vi "OPC_chk (SubVI).vi"(4 "error in":errorcluster, 7 "VISA in":refnum<visa-resource-name>) -> (0 "error out":errorcluster, 2 "opc?":bool, 3 "VISA out":refnum<visa-resource-name>)   [LabVIEW 2014]
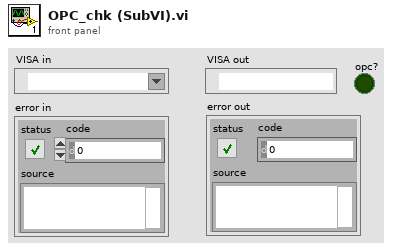
[diagram p1: front panel]
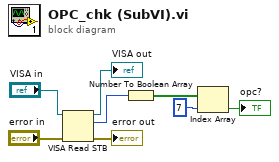
[diagram p0: block diagram]
diagram:
  n1 = VISA Read STB(8:"error in", 11:"VISA in") -> (0:→"error out":errorcluster, 2:w6:u16, 3:→"VISA out":refnum<visa-resource-name>)
  n2 = Number To Boolean Array(number=w6) -> (Boolean array=w7:bool[])
  n3 = Index Array(array=w7, index=7) -> (element=→"opc?":bool)
